vi "Scan for Measurements.vi"(8 "error in (no error)":errorcluster, 11 "Common Measurements in":refnum<class "Common Measurements.lvclass">) -> (0 "error out":errorcluster, 3 "Common Measurements out":refnum<class "Common Measurements.lvclass">)   [LabVIEW 2015, in "Common Measurements.lvclass"]
uses:
  Common Measurements.lvclass
  Measurement Timer/Measurement Timer.lvclass
  Common Measurements.lvclass/Common Measurements.ctl
  Mag Lab Measure Controller/Mag Lab Measure Controller.lvclass/Mag Lab Measure Controller.ctl
  Hardware/Mag Lab Hardware Function.ctl
  Mag Lab Root/Mag Lab Root.lvclass/Mag Lab Root.ctl
  Mag Lab Measure Base/Mag Lab Measure Base.lvclass/Mag Lab Measure Base.ctl
  Common Measurements Interface Messages/Select menu measurements Msg/Select menu measurements Msg.lvclass/Select menu measurements Msg.ctl
  <vilib>/ActorFramework/Message Enqueuer/Message Enqueuer.lvclass/Message Enqueuer.ctl
  <vilib>/ActorFramework/Message Enqueuer/Enqueue.vi
  <vilib>/ActorFramework/Message Priority Queue/Priority Enqueue.vi
  Mag Lab Measure Controller/Mag Lab Measure Controller.lvclass
  <vilib>/ActorFramework/Message Enqueuer/Message Enqueuer.lvclass
  Hardware/Mag Lab Hardware.lvclass
  Common Measurements Interface Messages/Select menu measurements Msg/Select menu measurements Msg.lvclass
  Mag Lab Measure Base/Mag Lab Measure Base.lvclass
  Mag Lab Error Handler/Mag Lab Error Handler.lvclass
  Thermopower/Termopower Measurement/Thermopower Measurement.lvclass
  Meter Measurement/Meter Measurement.lvclass
  Measurements/Sequencer Measurement/Sequencer Measurement.lvclass
  Mag Lab Root/Mag Lab Root.lvclass
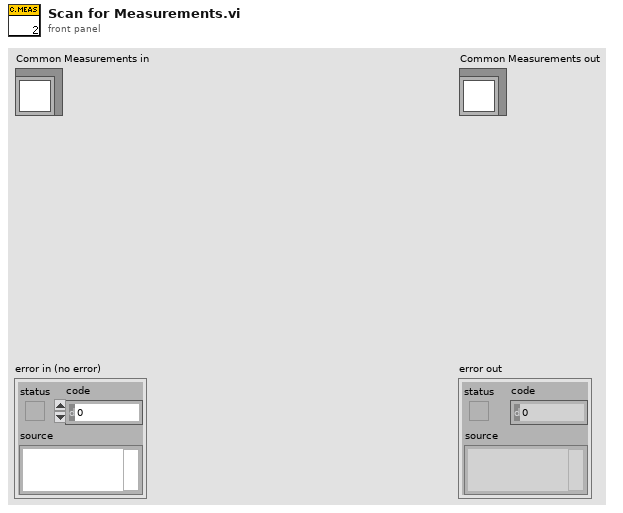
[diagram p1: front panel]
types:
  T1 = cluster{"Hardware Queue":refnum<class "Message Enqueuer.lvclass">, "HW Class":refnum<class "Mag Lab Hardware.lvclass">}[]
  T2 = typedef "Mag Lab Hardware Function.ctl" = enum16{"Input", "Voltmeter", "Output", "Current source", "Digitizer", "Temperature controller"}
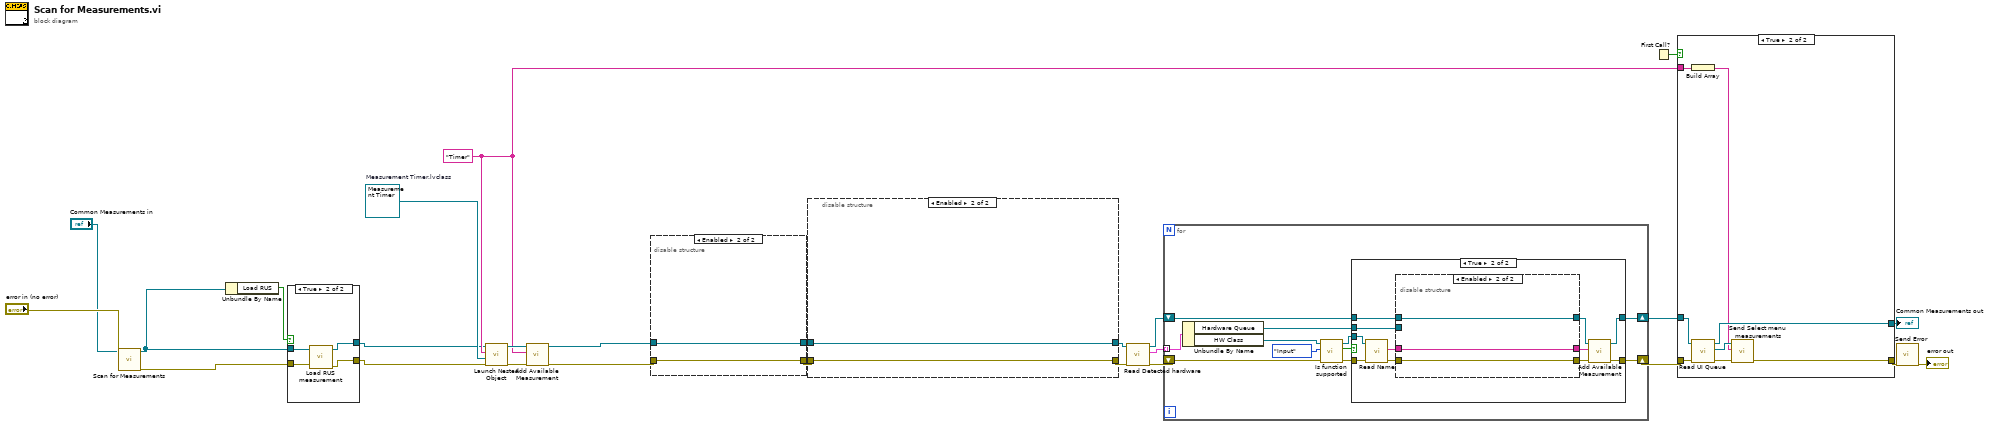
[diagram p0: block diagram]
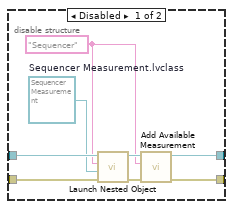
[diagram p3: hidden frame]
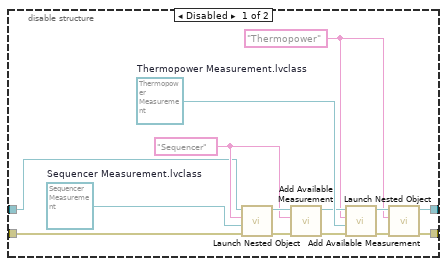
[diagram p4: hidden frame]
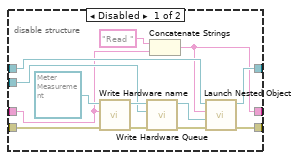
[diagram p7: hidden frame]
diagram:
  w10 = "Timer" ("Name")
  w20 = refnum<class "Measurement Timer.lvclass"> refnum  # Measurement Timer.lvclass
  n1 = call-parent "Scan for Measurements.vi"("error in (no error)"="error in (no error)", "Mag Lab Measure Controller in"="Common Measurements in") -> ("error out"=w5:errorcluster, "Mag Lab Measure Controller out"=w3:refnum<class "Common Measurements.lvclass">)  [unwired: 8 in]
  n2 = Unbundle By Name(w3) -> ("Load RUS"=w4:bool)
  n3 = case shown="True" w4 {
    tunnel: w5 -> [w28 w32]
    tunnel: w3 -> [w27 w31]
    tunnel: [w28 w30] -> w2
    tunnel: [w27 w29] -> w1
    frame False {
    }
    frame True {
      n4 = call "Load RUS measurement.vi"("error in (no error)"=w32, "Common Measurements in"=w31) -> ("error out"=w30:errorcluster, "Common Measurements out"=w29:refnum<class "Common Measurements.lvclass">)  [unwired: 8 in]
    }
  }
  n5 = call "Launch Nested Object.vi"("error in (no error)"=w2, "Object"=w20, "name"=w10, "Mag Lab Measure Base in"=w1) -> ("error out"=w18:errorcluster, "Mag Lab Measure Base out"=w17:refnum<class "Common Measurements.lvclass">)  [unwired: 5 in, 1 out]
  n6 = call-dynamic "Add Available Measurement.vi"("error in (no error)"=w18, "Name"=w10, "Common Measurements in"=w17) -> ("error out"=w7:errorcluster, "Common Measurements out"=w6:refnum<class "Common Measurements.lvclass">)  [unwired: 7 in]
  n7 = disable-structure shown="Enabled" {
    disable-tunnel: [w40 w41] -> w9
    disable-tunnel: [w39 w42] -> w8
    disable-tunnel: w7 -> [w38 w41]
    disable-tunnel: w6 -> [w36 w42]
    frame Disabled {
      w33 = "Sequencer" ("Name")
      w34 = refnum<class "Sequencer Measurement.lvclass"> refnum  # Sequencer Measurement.lvclass
      n8 = call "Launch Nested Object.vi"("error in (no error)"=w38, "Object"=w34, "name"=w33, "Mag Lab Measure Base in"=w36) -> ("error out"=w37:errorcluster, "Mag Lab Measure Base out"=w35:refnum<class "Common Measurements.lvclass">)  [unwired: 5 in, 1 out]
      n9 = call-dynamic "Add Available Measurement.vi"("error in (no error)"=w37, "Name"=w33, "Common Measurements in"=w35) -> ("error out"=w40:errorcluster, "Common Measurements out"=w39:refnum<class "Common Measurements.lvclass">)  [unwired: 7 in]
    }
    frame Enabled {
    }
  }
  n10 = disable-structure shown="Enabled" {
    disable-tunnel: [w47 w58] -> w19
    disable-tunnel: w8 -> [w45 w57]
    disable-tunnel: w9 -> [w44 w58]
    disable-tunnel: [w43 w57] -> w16
    frame Disabled {
      w53 = "Sequencer" ("name")
      w55 = refnum<class "Sequencer Measurement.lvclass"> refnum  # Sequencer Measurement.lvclass
      w56 = refnum<class "Thermopower Measurement.lvclass"> refnum  # Thermopower Measurement.lvclass
      w46 = "Thermopower" ("name")
      n11 = call "Launch Nested Object.vi"("error in (no error)"=w44, "Object"=w55, "name"=w53, "Mag Lab Measure Base in"=w45) -> ("error out"=w52:errorcluster, "Mag Lab Measure Base out"=w54:refnum<class "Common Measurements.lvclass">)  [unwired: 5 in, 1 out]
      n12 = call-dynamic "Add Available Measurement.vi"("error in (no error)"=w52, "Name"=w53, "Common Measurements in"=w54) -> ("error out"=w51:errorcluster, "Common Measurements out"=w50:refnum<class "Common Measurements.lvclass">)  [unwired: 7 in]
      n13 = call "Launch Nested Object.vi"("error in (no error)"=w51, "Object"=w56, "name"=w46, "Mag Lab Measure Base in"=w50) -> ("error out"=w49:errorcluster, "Mag Lab Measure Base out"=w48:refnum<class "Common Measurements.lvclass">)  [unwired: 5 in, 1 out]
      n14 = call-dynamic "Add Available Measurement.vi"("error in (no error)"=w49, "Name"=w46, "Common Measurements in"=w48) -> ("error out"=w47:errorcluster, "Common Measurements out"=w43:refnum<class "Common Measurements.lvclass">)  [unwired: 7 in]
    }
    frame Enabled {
    }
  }
  n15 = call "Read Detected hardware.vi"("error in (no error)"=w19, "Mag Lab Measure Controller in"=w16) -> ("error out"=w23:errorcluster, "Detected hardware"=w22:T1, "Mag Lab Measure Controller out"=w21:refnum<class "Common Measurements.lvclass">)  [unwired: 7 in]
  n16 = for {
    tunnel: w22 -> [w69] mode=indexing
    shift-right: [w64] -> w13
    shift-left: w23 -> [w67]
    shift-right: [w60] -> w14
    shift-left: w21 -> [w61]
    n17 = Unbundle By Name(w69) -> ("Hardware Queue"=w59:refnum<class "Message Enqueuer.lvclass">, "HW Class"=w68:refnum<class "Mag Lab Hardware.lvclass">)
    n18 = call-dynamic "Is function supported.vi"("error in (no error)"=w67, "Hardware function"=Mag_Lab_Hardware_Function."Input", "Mag Lab Hardware in"=w68) -> ("error out"=w65:errorcluster, "Supported"=w63:bool, "Mag Lab Hardware out"=w62:refnum<class "Mag Lab Hardware.lvclass">)  [unwired: 6 in]
    n19 = case shown="True" w63 {
      tunnel: w65 -> [w71 w81]
      tunnel: [w71 w75] -> w64
      tunnel: w62 -> [_ w82]
      tunnel: w61 -> [w70 w80]
      tunnel: [w70 w74] -> w60
      tunnel: w59 -> [_ w78]
      frame False {
      }
      frame True {
        n20 = call "Read Name.vi"("error in (no error)"=w81, "Mag Lab Root in"=w82) -> ("error out"=w79:errorcluster, "Name"=w73:string)  [unwired: 7 in, 1 out]
        n21 = disable-structure shown="Enabled" {
          disable-tunnel: w80 -> [w95 w98]
          disable-tunnel: w79 -> [w94 w96]
          disable-tunnel: w78 -> [w88 _]
          disable-tunnel: [w87 w98] -> w77
          disable-tunnel: [w86 w96] -> w76
          disable-tunnel: w73 -> [w85 w97]
          disable-tunnel: [w84 w97] -> w72
          frame Disabled {
            n22 = call "Write Hardware name.vi"("error in (no error)"=w94, "Hardware name"=w85, "Meter Measurement in"=refnum<class "Meter Measurement.lvclass"> refnum ("Meter Measurement.lvclass")) -> ("error out"=w92:errorcluster, "Meter Measurement out"=w91:refnum<class "Meter Measurement.lvclass">)  [unwired: 7 in]
            n23 = call "Write Hardware Queue.vi"("error in (no error)"=w92, "Actor Framework:Message Enqueuer"=w88, "Meter Measurement in"=w91) -> ("error out"=w89:errorcluster, "Meter Measurement out"=w90:refnum<class "Meter Measurement.lvclass">)  [unwired: 7 in]
            n24 = Concatenate Strings("Read " ("string"), w85) -> (w84:string)
            n25 = call "Launch Nested Object.vi"("error in (no error)"=w89, "Object"=w90, "name"=w84, "Mag Lab Measure Base in"=w95) -> ("error out"=w86:errorcluster, "Mag Lab Measure Base out"=w87:refnum<class "Common Measurements.lvclass">)  [unwired: 5 in, 1 out]
          }
          frame Enabled {
          }
        }
        n26 = call-dynamic "Add Available Measurement.vi"("error in (no error)"=w76, "Name"=w72, "Common Measurements in"=w77) -> ("error out"=w75:errorcluster, "Common Measurements out"=w74:refnum<class "Common Measurements.lvclass">)  [unwired: 7 in]
      }
    }
  }
  n27 = First Call?() -> (First Call?: T/F=w15:bool)
  n28 = case shown="True" w15 {
    tunnel: w14 -> [w100 w108]
    tunnel: w13 -> [w99 w107]
    tunnel: [w99 w106] -> w12
    tunnel: [w100 w104] -> w11
    tunnel: w10 -> [_ w102]
    frame False {
    }
    frame True {
      n29 = Build Array(w102) -> (w101:string[])
      n30 = call "Read UI Queue.vi"("error in (no error)"=w107, "Mag Lab Measure Base in"=w108) -> ("error out"=w105:errorcluster, "Actor Framework.lvlib:Message Enqueuer"=w103:refnum<class "Message Enqueuer.lvclass">, "Mag Lab Measure Base out"=w104:refnum<class "Common Measurements.lvclass">)  [unwired: 7 in]
      n31 = call "Send Select menu measurements.vi"("error in (no error)"=w105, "Measurements"=w101, "Message Enqueuer"=w103) -> ("error out"=w106:errorcluster)  [unwired: 7 in, 1 out]
    }
  }
  "Common Measurements out" <- w11
  n32 = call "Send Error.vi"("error in (no error)"=w12) -> ("error out"=→"error out":errorcluster)  [unwired: 9 in, 1 out]
